vi "Common.vi"(10 "xData in":refnum<class "xData.lvclass">, 11 "Controller in":refnum<class "Controller.lvclass">) -> ()   [LabVIEW 2014, in "Controller.lvlib" / "Controller.lvclass"]
uses:
  Controller.lvclass
  Data/xData.lvclass
  <vilib>/Platform/TimedLoop/XDataNode/timing_clust.ctl
  <vilib>/Platform/TimedLoop/XDataNode/nitl_modes.ctl
  <vilib>/Platform/TimedLoop/XDataNode/wakeup.ctl
  Controller.lvclass/Controller.ctl
  SuperActor/Ex Nested.lvclass/Ex Nested.ctl
  <vilib>/ActorFramework/Actor/Actor.lvclass/Actor.ctl
  <vilib>/ActorFramework/Message Enqueuer/Message Enqueuer.lvclass/Message Enqueuer.ctl
  Update Controller Data MSG.lvclass
  reusable/Switch/Switch.lvclass/Switch.ctl
  Data/xData.lvclass/xData.ctl
  reusable/Data/Data.lvclass/Data.ctl
  reusable/DAQ Device/Device/Generic Data Update Data MSG/Generic Update Data Message.lvclass/Generic Update Data Message.ctl
  <vilib>/DAQmx/write.llb/DAQmx Write (Digital Bool 1Line 1Point).vi
  <vilib>/DAQmx/read.llb/DAQmx Read (Digital 1D Bool NChan 1Samp 1Line).vi
  <vilib>/DAQmx/read.llb/DAQmx Read (Analog 1D DBL 1Chan NSamp).vi
  <vilib>/Analysis/baseanly.llb/Mean (DBL).vi
  reusable/Switch/Read LastSwitch.vi
  Data/Write Cabin.vi
  Data/Write Filter.vi
  Data/Write Interlock.vi
  Data/Write PumpBlocked.vi
  Data/Write fCycle.vi
  Data/Write ImpDiffV.vi
  Data/Write SysMsg.vi
  reusable/Data/Write write time.vi
  reusable/DAQ Device/Device/Generic Data Update Data MSG/Write ID.vi
  reusable/DAQ Device/Device/Generic Data Update Data MSG/Write Data.vi
  Accessors/Read Switch DVR.vi
  SuperActor/Read Log Session.vi
  <vilib>/ActorFramework/Message Enqueuer/Init from Existing Queue.vi
  <vilib>/DAQmx/miscellaneous.llb/DAQmx Fill In Error Info.vi
  reusable/Switch/Read maxElapsedTime.vi
  reusable/Data/Write measTime.vi
  <vilib>/ActorFramework/Message Priority Queue/Priority Enqueue.vi
  <vilib>/ActorFramework/Message Enqueuer/Message Enqueuer.lvclass
  reusable/Switch/Switch.lvclass
  <userlib>/_Session Fwk/Session - Root.lvclass
  <vilib>/Platform/TimedLoop/XDataNode/XDataNode.xnode
  <vilib>/ActorFramework/Actor/Actor.lvclass
  reusable/Session APIs/Session Log/System Log.lvclass
  <vilib>/Analysis/NI_AALBase.lvlib
  <vilib>/Platform/TimedLoop/XDataNode/XDNodeRunTimeDep.lvlib
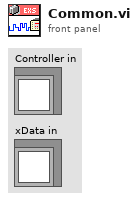
[diagram p1: front panel]
types:
  T1 = typedef "Session - Root.lvclass/Session Handle.ctl" = refnum<data-value>
  T2 = typedef "XDNodeRunTimeDep.lvlib/timing_clust.ctl" = cluster{"Expected End [f-1]":u64, "Actual End [f-1]":u64, "Finished Late? [f-1]":bool, "Expected End [i-1]":u64, "Actual End [i-1]":u64, "Finished Late? [i-1]":bool, "Expected Start [i]":u64, "Actual Start [i]":u64, "Expected Start [f]":u64, "Actual Start [f]":u64, "Source Name":string, "Structure Name":string, "Period":i64, "Deadline":i64, "Offset":i64, "Start":i64, "Priority":i32, "Timeout":i32, "Mode":T3, "Wakeup Reason":T4, "Error":errorcluster, "Source Type":string, "Secondary Source Type":string, "Global End Time":u64, "Global Start Time":u64, "Frame Duration":u64, "Iteration Duration":u64, "Assigned CPU":i32, "I/O Scan Engine Mode":u32}
  T3 = typedef "XDNodeRunTimeDep.lvlib/nitl_modes.ctl" = enum32{"No Change", "Process missed periods, maintain original phase", "Discard missed periods, maintain original phase", "Process missed periods, ignore original phase", "Discard missed periods, ignore original phase"}
  T4 = typedef "XDNodeRunTimeDep.lvlib/wakeup.ctl" = enum32{"Normal", "Aborted", "Asynchronous wakeup", "Timing source error", "Timed loop error", "Timeout"}
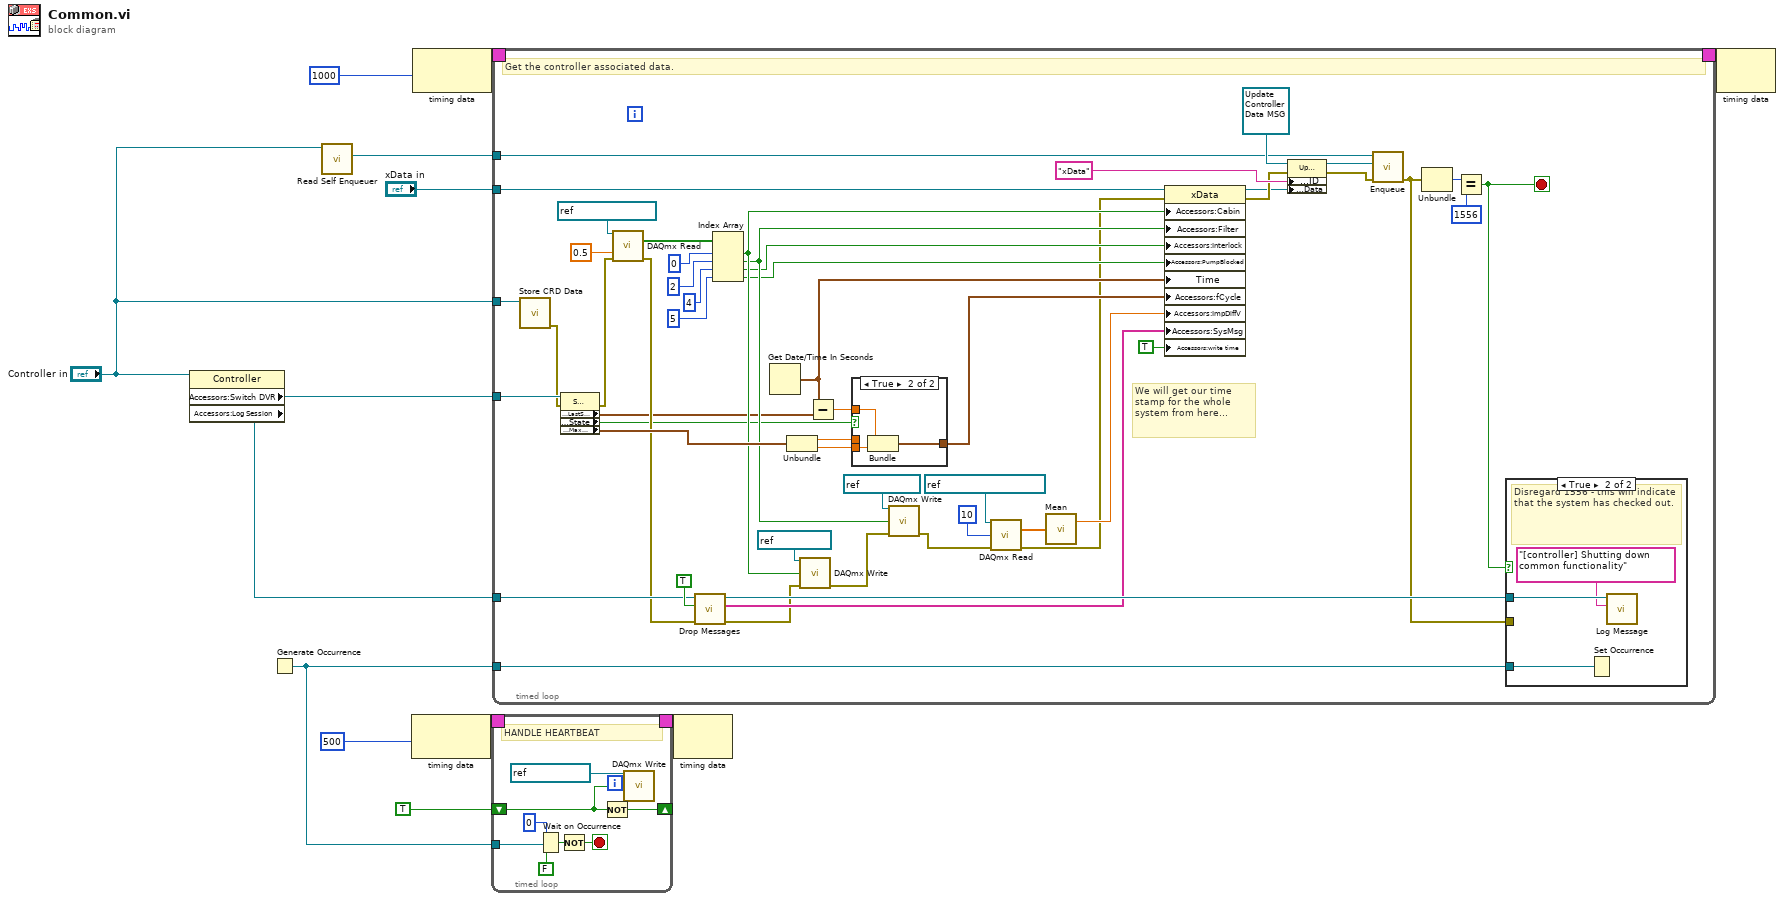
[diagram p0: block diagram]
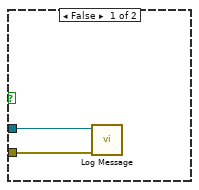
[diagram p2: hidden frame]
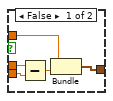
[diagram p3: hidden frame]
diagram:
  n1 = property class="Controller"(reference="Controller in") -> ("Accessors:Switch DVR"=w2:refnum<data-value>, "Accessors:Log Session"=w1:T1)  [unwired: 1 in, 2 out]
  n2 = Generate Occurrence() -> (w4:refnum<k4>)
  n3 = call <vilib>:"Read Self Enqueuer.vi"("Actor"="Controller in") -> ("Self Enqueuer"=w12:refnum<class "Message Enqueuer.lvclass">)  [unwired: 10 in]
  n4 = node-c288(i64 500 ("Period")) -> (w7:T2)
  n5 = node-c288(i64 1000 ("millisecond multiple")) -> (w11:T2)
  n6 = timed-loop {
    shift-right: [w20] -> _
    shift-left: TRUE -> [w21]
    timing: w7 -> [_]
    timing-out: [_] -> w6
    tunnel: w4 -> [w18]
    stop <- w15 stop-if-true
    # "HANDLE HEARTBEAT"
    n7 = Wait on Occurrence(1:FALSE ("ignore previous (T)"), 2:w18, 3:0 ("ms timeout (-1)")) -> (0:w16:bool)
    n8 = Not(x=w16) -> (.not. x?=w15:bool)
    n9 = Not(x=w21) -> (.not. x?=w20:bool)
    n10 = call-poly <vilib>:"DAQmx Write.vi"("task/channels in"=refnum<k21> "Heartbeat", "data"=w21) -> ()  [unwired: 11 in, 3 out]
  }
  n11 = timed-loop {
    tunnel: "xData in" -> [w64]
    tunnel: w12 -> [w65]
    tunnel: w1 -> [w62]
    tunnel: w2 -> [w61]
    tunnel: "Controller in" -> [w51]
    timing: w11 -> [_]
    timing-out: [_] -> w10
    tunnel: w4 -> [w24]
    stop <- w28 stop-if-true
    # "We will get our time stamp for the whole system from here..."
    # "Get the controller associated data."
    n12 = call "Store CRD Data.vi"("Controller in"=w51) -> ("error out"=w39:errorcluster)  [unwired: 9 in, 1 out]
    n13 = property class="Switch"(reference=w61, error in=w39) -> (error out=w38:errorcluster, "Accessors:LastSwitch"=w25:timestamp, "Data Access:State"=w26:bool, "Data Access:Max Elapsed Time"=w60:cluster{"Period":sgl, "Length":sgl})  [unwired: 1 out]
    n14 = call-poly <vilib>:"DAQmx Read.vi"("task/channels in"=refnum<k21> "General Input", "timeout"=0.5, "error in"=w38) -> ("data"=w71:bool[], "error out"=w30:errorcluster)  [unwired: 10 in, 1 out]
    n15 = call "Drop Messages.vi"("error in"=w30, "Drop?"=TRUE, "log in"=w62) -> ("error out"=w29:errorcluster, "Current Msgs"=w34:string[], "log out"=w53:T1)  [unwired: 6 in]
    n16 = Index Array(array=w71, index #1=0 ("index"), index #2=2 ("index"), index #3=4 ("index"), index #4=5 ("index")) -> (element #1=w49:bool, element #2=w47:bool, element #3=w41:bool, element #4=w40:bool)
    n17 = Get Date/Time In Seconds() -> (seconds since 1Jan1904=w59:timestamp)
    n18 = Unbundle(w60) -> ("Period"=w56:sgl, "Length"=w57:sgl)
    n19 = call-poly <vilib>:"DAQmx Write.vi"("task/channels in"=refnum<k21> "Inlet LED", "data"=w49, "error in"=w29) -> ("error out"=w37:errorcluster)  [unwired: 10 in, 2 out]
    n20 = Subtract(x=w59, y=w25) -> (x-y=w58:dbl)
    n21 = case shown="True" w26 {
      tunnel: w58 -> [w85 w88]
      tunnel: w57 -> [w84 w87]
      tunnel: w56 -> [w83 _]
      tunnel: [w81 w86] -> w55
      frame False {
        n22 = Subtract(x=w83, y=w84) -> (x-y=w82:sgl)
        n23 = Bundle(w85, w82) -> (w81:cluster{dbl, sgl})  [unwired: 1 in]
      }
      frame True {
        n24 = Bundle(w88, "Length"=w87) -> (w86:cluster{dbl, "Length":sgl})  [unwired: 1 in]
      }
    }
    n25 = call-poly <vilib>:"DAQmx Write.vi"("task/channels in"=refnum<k21> "Filter LED", "data"=w47, "error in"=w37) -> ("error out"=w36:errorcluster)  [unwired: 10 in, 2 out]
    n26 = call-poly <vilib>:"DAQmx Read.vi"("task/channels in"=refnum<k21> "Blocked Impactor", "number of samples per channel"=10, "error in"=w36) -> ("data"=w44:dbl[], "error out"=w35:errorcluster)  [unwired: 10 in, 1 out]
    n27 = call-poly <vilib>:"Mean.vi"("X"=w44) -> ("mean"=w42:dbl)  [unwired: 1 out]
    n28 = property class="xData"(reference=w64, error in=w35, "Accessors:Cabin"=w49, "Accessors:Filter"=w47, "Accessors:Interlock"=w41, "Accessors:PumpBlocked"=w40, "Time"=w59, "Accessors:fCycle"=w55, "Accessors:ImpDiffV"=w42, "Accessors:SysMsg"=w34, "Accessors:write time"=TRUE ("write time")) -> (reference out=w67:refnum<class "xData.lvclass">, error out=w68:errorcluster)
    n29 = property class="Update Data MSG"(reference=refnum<class "Update Controller Data MSG.lvclass"> refnum ("Controller.lvlib:Update Data MSG"), error in=w68, "Accessors:ID"="xData" ("ID"), "Accessors:Data"=w67) -> (reference out=w66:refnum<class "Update Controller Data MSG.lvclass">, error out=w52:errorcluster)
    n30 = call <vilib>:"Enqueue.vi"("error in (no error)"=w52, "Message"=w66, "Message Enqueuer in"=w65) -> ("error out"=w27:errorcluster)  [unwired: 7 in, 1 out]
    n31 = Unbundle(w27) -> ("code"=w32:i32)  [unwired: 2 out]
    n32 = Equal?(x=w32, y=1556) -> (x = y?=w28:bool)
    n33 = case shown="True" w28 {
      tunnel: w53 -> [w77 w80]
      tunnel: w27 -> [w76 _]
      tunnel: w24 -> [_ w78]
      frame False {
        n34 = call "Log Message.vi"("error in"=w76, "session in"=w77) -> ()  [unwired: 8 in, 2 out]
      }
      frame True {
        # "Disregard 1556 - this will indicate that the system has checked out."
        n35 = Set Occurrence(w78) -> ()
        n36 = call "Log Message.vi"("MSG In"="[controller] Shutting down common functionality", "session in"=w80) -> ()  [unwired: 8 in, 2 out]
      }
    }
  }
  n37 = node-c288(w6) -> ()  [unwired: 1 out]
  n38 = node-c288(w10) -> ()  [unwired: 1 out]
